vi "SelfTerminate.vi"(8 "error in (no error)":errorcluster, 11 "SMO in":refnum<class "SMO.lvclass">) -> (0 "error out":errorcluster, 3 "SMO out":refnum<class "SMO.lvclass">)   [LabVIEW 2013, in "SMO.lvclass"]
uses:
  SMO.lvclass
  SMO.lvclass/SMO.ctl
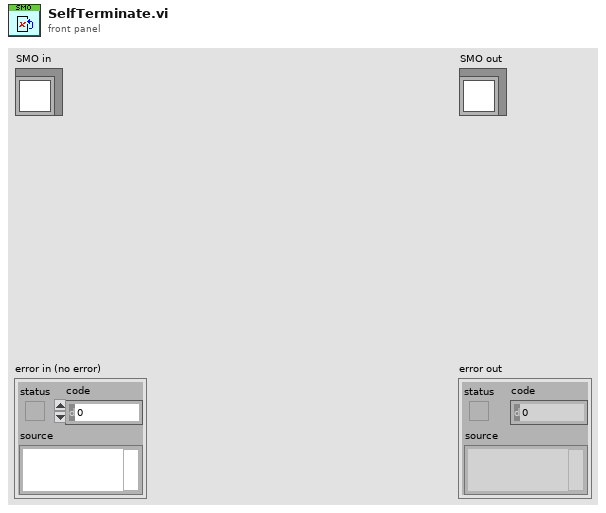
[diagram p1: front panel]
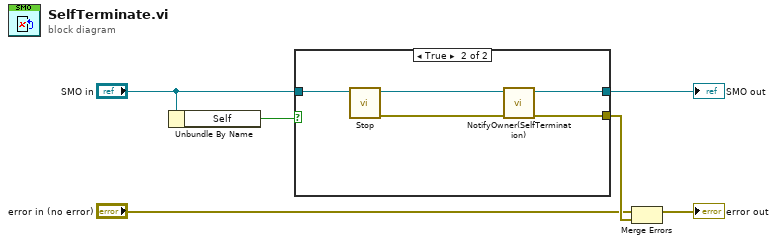
[diagram p0: block diagram]
diagram:
  n1 = Unbundle By Name("SMO in") -> ("Self"=w6:bool)
  n2 = case shown="True" w6 {
    tunnel: "SMO in" -> [w7 w12]
    tunnel: [w7 w10] -> w4
    tunnel: [_ w8] -> w3
    frame False {
    }
    frame True {
      n3 = call "Stop.vi"("SMO"=w12) -> ("error out"=w9:errorcluster, "SMO out"=w11:refnum<class "SMO.lvclass">)  [unwired: 9 in]
      n4 = call "NotifyOwner(SelfTermination).vi"("error in (no error)"=w9, "SMO in"=w11) -> ("error out"=w8:errorcluster, "SMO out"=w10:refnum<class "SMO.lvclass">)  [unwired: 8 in]
    }
  }
  "SMO out" <- w4
  n5 = Merge Errors("error in (no error)", w3) -> (→"error out":errorcluster)
